vi "Save_Default_Project_Reference.vi"(1 "error in":errorcluster) -> (0 "error out":errorcluster)   [LabVIEW 2021]
uses:
  <vilib>/Utility/config.llb/Write Key (String).vi
  <vilib>/Utility/config.llb/NI_LVConfig.lvlib
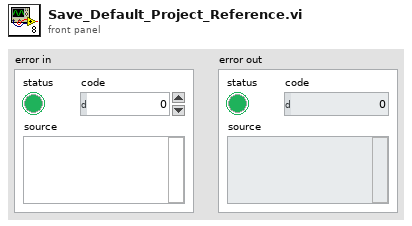
[diagram p1: front panel]
types:
  T1 = typedef "NI_LVConfig.lvlib/Config Data RefNum.ctl" = refnum<k1>
  T2 = cluster{"VI Name":string, "String Path":string}[]
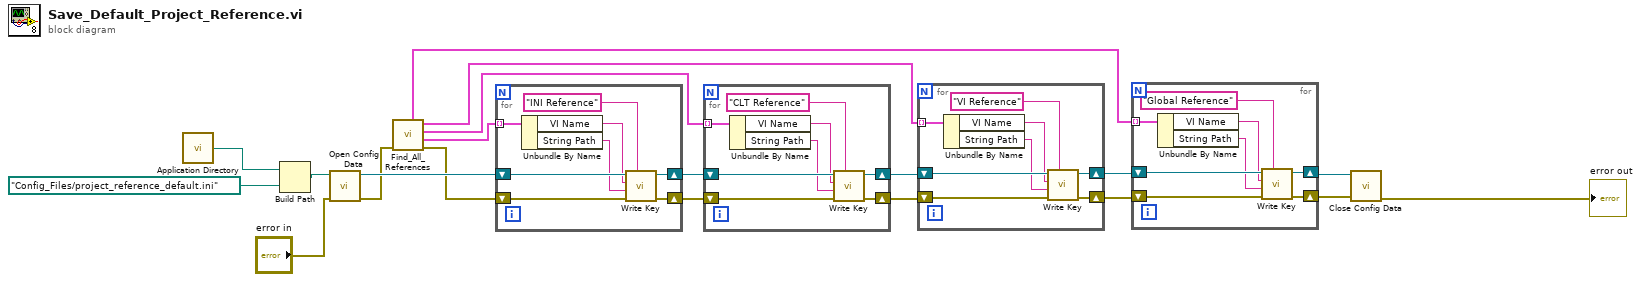
[diagram p0: block diagram]
diagram:
  n1 = call <vilib>:"Application Directory.vi"() -> ("Application Directory"=w3:path)
  n2 = Build Path(base path=w3, name or relative path=path "Config_Files/project_reference_default.ini" ("configuration file path")) -> (appended path=w4:path)
  n3 = call <vilib>:"Open Config Data.vi"("error in (no error)"="error in", "configuration file path"=w4) -> ("error out"=w11:errorcluster, "refnum"=w20:T1)  [unwired: 7 in, 1 out]
  n4 = call "Find_All_References.vi"("error in"=w11) -> ("error out"=w10:errorcluster, "INI References"=w6:T2, "CTL References"=w7:T2, "VI References"=w8:T2, "Global References"=w9:T2)  [unwired: 4 in]
  n5 = for {
    shift-right: [w28] -> w19
    shift-left: w20 -> [w26]
    shift-right: [w27] -> w18
    shift-left: w10 -> [w25]
    tunnel: w6 -> [w23] mode=indexing
    n6 = Unbundle By Name(w23) -> ("VI Name"=w24:string, "String Path"=w22:string)
    n7 = call-poly <vilib>:"Write Key.vi"("section"="INI Reference", "error in (no error)"=w25, "value"=w22, "key"=w24, "refnum"=w26) -> ("error out"=w27:errorcluster, "refnum out"=w28:T1)  [unwired: 4 in, 1 out]
  }
  n8 = for {
    shift-right: [w36] -> w17
    shift-left: w19 -> [w34]
    shift-right: [w35] -> w16
    shift-left: w18 -> [w33]
    tunnel: w7 -> [w31] mode=indexing
    n9 = Unbundle By Name(w31) -> ("VI Name"=w32:string, "String Path"=w30:string)
    n10 = call-poly <vilib>:"Write Key.vi"("section"="CLT Reference", "error in (no error)"=w33, "value"=w30, "key"=w32, "refnum"=w34) -> ("error out"=w35:errorcluster, "refnum out"=w36:T1)  [unwired: 4 in, 1 out]
  }
  n11 = for {
    shift-right: [w44] -> w15
    shift-left: w17 -> [w42]
    shift-right: [w43] -> w14
    shift-left: w16 -> [w41]
    tunnel: w8 -> [w39] mode=indexing
    n12 = Unbundle By Name(w39) -> ("VI Name"=w40:string, "String Path"=w38:string)
    n13 = call-poly <vilib>:"Write Key.vi"("section"="VI Reference", "error in (no error)"=w41, "value"=w38, "key"=w40, "refnum"=w42) -> ("error out"=w43:errorcluster, "refnum out"=w44:T1)  [unwired: 4 in, 1 out]
  }
  n14 = for {
    shift-right: [w52] -> w12
    shift-left: w15 -> [w50]
    shift-right: [w51] -> w13
    shift-left: w14 -> [w49]
    tunnel: w9 -> [w47] mode=indexing
    n15 = Unbundle By Name(w47) -> ("VI Name"=w48:string, "String Path"=w46:string)
    n16 = call-poly <vilib>:"Write Key.vi"("section"="Global Reference", "error in (no error)"=w49, "value"=w46, "key"=w48, "refnum"=w50) -> ("error out"=w51:errorcluster, "refnum out"=w52:T1)  [unwired: 4 in, 1 out]
  }
  n17 = call <vilib>:"Close Config Data.vi"("error in (no error)"=w13, "refnum"=w12) -> ("error out"=→"error out":errorcluster)  [unwired: 8 in, 1 out]
